vi "LJ_Open.vi"(8 "error in":errorcluster, 11 "DeviceType":string="LJM_dtTSERIES") -> (0 "error out":errorcluster, 2 "Success?":bool, 3 "Handle Out":i32)   [LabVIEW 2020]
panel:
  out "ConnectionType":i32
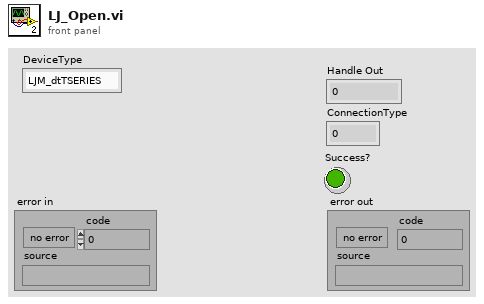
[diagram p1: front panel]
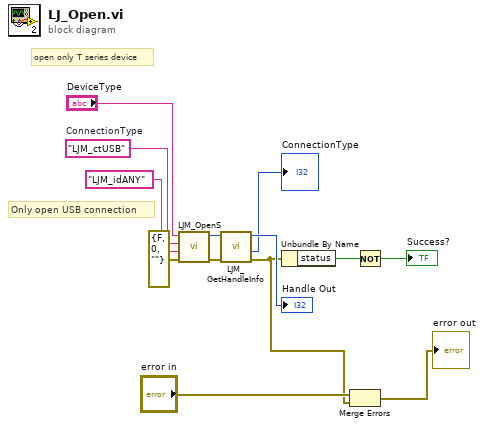
[diagram p0: block diagram]
diagram:
  w11 = "LJM_ctUSB"  # ConnectionType
  # "Only open USB connection"
  # "open only T series device"
  n1 = call "LJM_OpenS.vi"("error in"=errorcluster {"status"=FALSE, "code"=0, "source"=""}, "Identifier"="LJM_idANY", "ConnectionType"=w11, "DeviceType"="DeviceType") -> ("error out"=w12:errorcluster, "Handle"=w13:i32)  [unwired: 6 in]
  n2 = call "LJM_GetHandleInfo.vi"("error in"=w12, "Handle In"=w13) -> ("error out"=w3:errorcluster, "ConnectionType"=→"ConnectionType":i32, "Handle Out"=→"Handle Out":i32)  [unwired: 2 in, 5 out]
  n3 = Unbundle By Name(w3) -> ("status"=w7:bool)
  n4 = Merge Errors("error in", w3) -> (→"error out":errorcluster)
  n5 = Not(x=w7) -> (.not. x?=→"Success?":bool)
